vi "XControl with Static Path Selector.vi"() -> ()   [LabVIEW 2016]
uses:
  <userlib>/_MGI/User Interface/Path Selector XControl/Class Hierarchy/Static File Selector/MGI Static Path Selector.lvclass
  <userlib>/_MGI/User Interface/Path Selector XControl/MGI Path Selector.xctl
  C:/Program Files (x86)/National Instruments/LabVIEW 2016/user.lib/_MGI/User Interface/Path Selector XControl/Class Hierarchy/MGI Path Selector.lvclass
panel:
  in  "Path Selector":path(xcontrol)
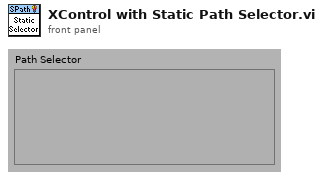
[diagram p1: front panel]
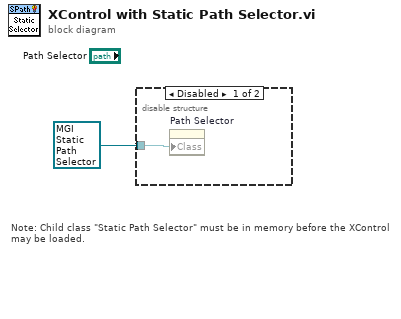
[diagram p0: block diagram]
diagram:
  # "Note: Child class \"Static Path Selector\" must be in memory before the XControl may be loaded."
  n1 = disable-structure shown="Disabled" {
    disable-tunnel: refnum<class "MGI Static Path Selector.lvclass"> refnum ("Static Path Selector.lvclass") -> [w2 _]
    frame Disabled {
      n2 = property on="Path Selector"("Class"=w2) -> ()  [unwired: 2 in, 2 out]
    }
    frame Enabled {
    }
  }
